vi "WPI_SPIBusCache.vi"(7 "Operation":T2, 8 "error in (no error)":errorcluster, 11 "SPI Bus":T1) -> (0 "error out":errorcluster, 2 "Allocated?":bool, 3 "SPI Bus Allocated":T1)   [LabVIEW 2017]
doc: "This software is licensed. Open the labview\\readme\\WPI Robotics Library Open Source License.txt file for more information."
uses:
  <vilib>/Rock Robotics/WPI/SPI/WPI_SPIBusCacheOp.ctl
  <vilib>/Rock Robotics/SystemInterfaces/spilib/spi_bus.ctl
  <vilib>/Rock Robotics/WPI/PWM/WPI_PWMChannelCacheOp.ctl
  <vilib>/Rock Robotics/WPI/MXP/WPI_MXP SPI Bus to first MXP Pin.vi
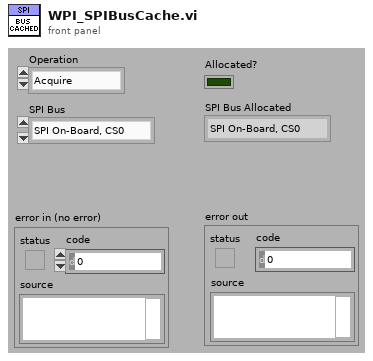
[diagram p1: front panel]
types:
  T1 = typedef "spi_bus.ctl" = enum16{"SPI On-Board, CS0", "SPI On-Board, CS1", "SPI On-Board, CS2", "SPI On-Board, CS3", "SPI MXP", "Invalid"}
  T2 = typedef "WPI_SPIBusCacheOp.ctl" = enum16{"Acquire", "Release", "Status"}
  T3 = typedef "WPI_PWMChannelCacheOp.ctl" = enum16{"Acquire", "Release", "Status"}
  T4 = typedef "WPI_MXP Shared MXP Pin.ctl" = enum16{"11", "13", "15", "17", "19", "21", "23", "25", "27", "29", "31", "18", "22", "26", "32", "34", "Invalid"}
  T5 = typedef "Semaphore RefNum" = refnum<k1>
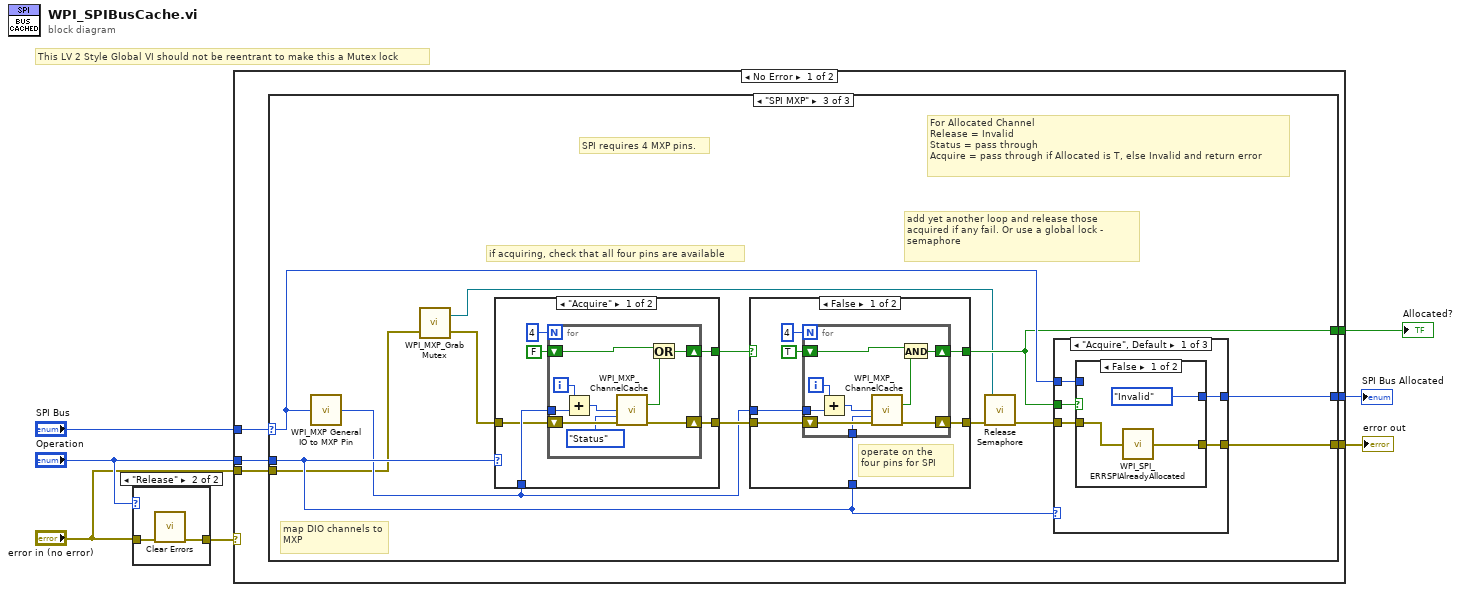
[diagram p0: block diagram]
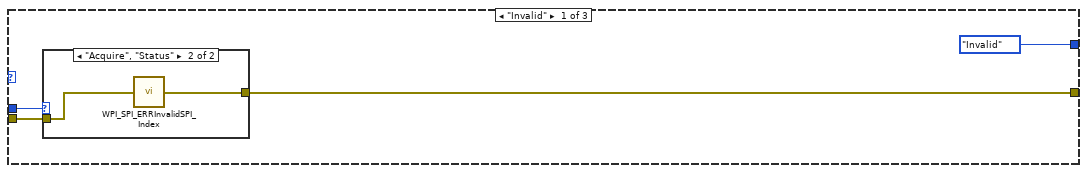
[diagram p3: hidden frame]
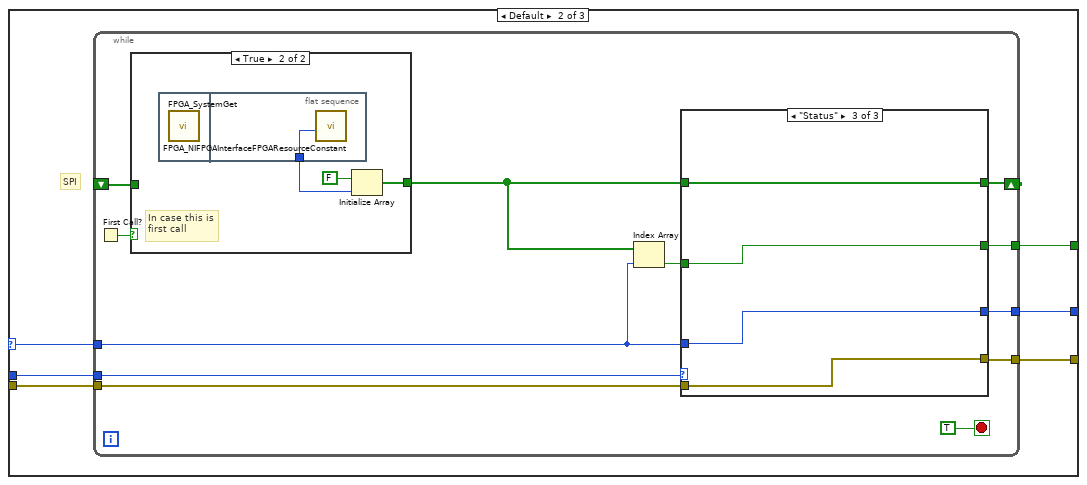
[diagram p5: hidden frame]
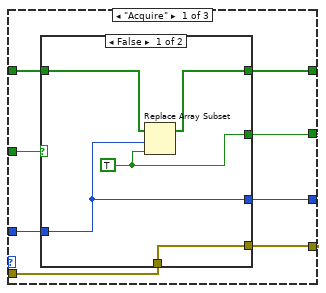
[diagram p6: hidden frame]
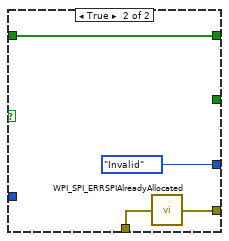
[diagram p7: hidden frame]
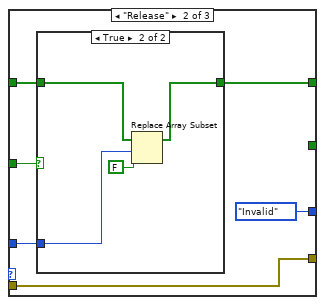
[diagram p8: hidden frame]
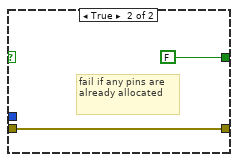
[diagram p11: hidden frame]
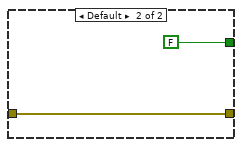
[diagram p12: hidden frame]
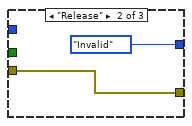
[diagram p14: hidden frame]
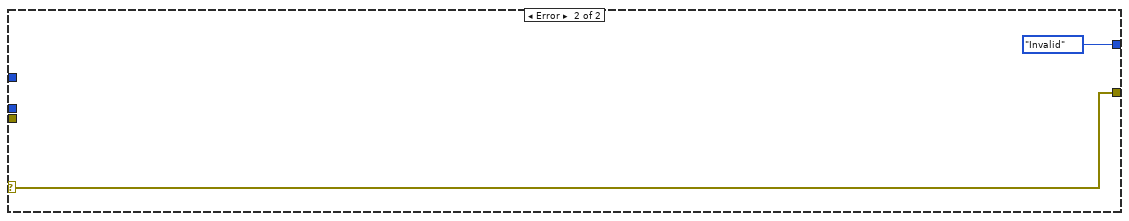
[diagram p16: hidden frame]
diagram:
  # "This LV 2 Style Global VI should not be reentrant to make this a Mutex lock"
  n1 = case shown="\"Release\"" "Operation" {
    tunnel: "error in (no error)" -> [w8 w10]
    tunnel: [w8 w9] -> w4
    frame "Acquire", Default {
    }
    frame "Release" {
      n2 = call <vilib>:"Clear Errors.vi"("error in (no error)"=w10) -> ("error out"=w9:errorcluster)  [unwired: 1 in, 5 out]
    }
  }
  n3 = case shown="No Error" w4 {
    selector: w4 -> [_ w142]
    tunnel: "Operation" -> [w16 _]
    tunnel: "SPI Bus" -> [w15 _]
    tunnel: [w14 w142] -> w1
    tunnel: [w13 _] -> w6
    tunnel: [w12 spi_bus."Invalid" ("SPI Bus")] -> w3
    tunnel: "error in (no error)" -> [w11 _]
    frame No Error {
      n4 = case shown="\"SPI MXP\"" w15 {
        selector: w15 -> [_ w25 w89]
        tunnel: w16 -> [w20 w29 w86]
        tunnel: [w19 w28 w91] -> w14
        tunnel: [_ w27 w85] -> w13
        tunnel: [spi_bus."Invalid" ("SPI Bus") w26 w90] -> w12
        tunnel: w11 -> [w18 w24 w79]
        frame "Invalid" {
          n5 = case shown="\"Acquire\", \"Status\"" w20 {
            tunnel: [w21 w23] -> w19
            tunnel: w18 -> [w21 w22]
            frame "Release" {
            }
            frame "Acquire", "Status" {
              n6 = call <vilib>:"WPI_SPI_ERRInvalidSPI_Index.vi"("error in (no error)"=w22) -> ("error out"=w23:errorcluster)
            }
          }
        }
        frame Default {
          # "SPI"
          n7 = while {
            shift-right: [w38] -> _
            shift-left: _ -> [w40]
            tunnel: w29 -> [w39]
            tunnel: w25 -> [w34]
            tunnel: [w37] -> w28
            tunnel: [w36] -> w27
            tunnel: [w33] -> w26
            tunnel: w24 -> [w31]
            stop <- TRUE stop-if-true
            n8 = First Call?() -> (First Call?: T/F=w41:bool)
            n9 = case shown="True" w41 {
              tunnel: w40 -> [w74 _]
              tunnel: [w74 w77] -> w35
              frame False {
              }
              frame True {
                # "In case this is\nfirst call"
                n10 = flat-sequence {
                  tunnel: [w78] -> w75
                  frame #0 {
                    n11 = call <vilib>:"FPGA_SystemGet.vi"() -> ()  [unwired: 11 in, 1 out]
                  }
                  frame #1 {
                    n12 = call <vilib>:"FPGA_NIFPGAInterfaceFPGAResourceConstant.vi"() -> ("NumberOfSPI"=w78:i32)  [unwired: 11 out]
                  }
                }
                n13 = Initialize Array(FALSE, w75) -> (w77:bool[])
              }
            }
            n14 = Index Array(array=w35, index=w34) -> (element=w30:bool)
            n15 = case shown="\"Status\"" w39 {
              tunnel: w35 -> [w45 w64 w73]
              tunnel: [w49 w62 w73] -> w38
              tunnel: w34 -> [w48 w63 w71]
              tunnel: [w47 w60 w70] -> w37
              tunnel: [w46 _ w72] -> w36
              tunnel: w30 -> [w44 w61 w72]
              tunnel: [w43 spi_bus."Invalid" ("SPI Bus") w71] -> w33
              tunnel: w31 -> [w42 w60 w70]
              frame "Acquire" {
                n16 = case shown="False" w44 {
                  tunnel: w45 -> [w53 w58]
                  tunnel: [w52 w58] -> w49
                  tunnel: w48 -> [w51 _]
                  tunnel: [w50 w57] -> w47
                  tunnel: [w54 _] -> w46
                  tunnel: [w51 spi_bus."Invalid" ("SPI Bus")] -> w43
                  tunnel: w42 -> [w50 w56]
                  frame False {
                    w54 = TRUE ("new element/subarray")
                    n17 = Replace Array Subset(array=w53, new element=w54, index=w51) -> (w52:bool[])
                  }
                  frame True {
                    n18 = call <vilib>:"WPI_SPI_ERRSPIAlreadyAllocated.vi"("error in (no error)"=w56) -> ("error out"=w57:errorcluster)
                  }
                }
              }
              frame "Release" {
                n19 = case shown="True" w61 {
                  tunnel: w64 -> [w65 w69]
                  tunnel: w63 -> [_ w68]
                  tunnel: [w65 w67] -> w62
                  frame False {
                  }
                  frame True {
                    n20 = Replace Array Subset(array=w69, new element=FALSE ("new element/subarray"), index=w68) -> (w67:bool[])
                  }
                }
              }
              frame "Status" {
              }
            }
          }
        }
        frame "SPI MXP" {
          # "add yet another loop and release those acquired if any fail. Or use a global lock - semaphore"
          # "SPI requires 4 MXP pins."
          # "if acquiring, check that all four pins are available"
          # "map DIO channels to MXP"
          # "For Allocated Channel\nRelease = Invalid\nStatus = pass through\nAcquire = pass through if Allocated is T, else Invalid and return error"
          n21 = call-poly <vilib>:"WPI_MXP General IO to MXP Pin.vi"("SPI Bus"=w89) -> ("Shared MXP Pin"=w82:T4)  [unwired: 14 in]
          n22 = call <vilib>:"WPI_MXP_Grab Mutex.vi"("error in"=w79) -> ("error out"=w80:errorcluster, "semaphore out"=w81:T5)  [unwired: 1 in]
          n23 = case shown="\"Acquire\"" w86 {
            tunnel: [w115 w126] -> w88
            tunnel: w82 -> [w114 _]
            tunnel: w80 -> [w113 w126]
            tunnel: [w110 FALSE] -> w87
            frame "Acquire" {
              n24 = for {
                N: 4 -> [_]
                tunnel: w114 -> [w123]
                shift-right: [w124] -> w115
                shift-left: w113 -> [w122]
                shift-right: [w119] -> w110
                shift-left: FALSE -> [w118]
                i -> [w120]
                n25 = Add(x=w120, y=w123) -> (x+y=w121:i32)
                n26 = call <vilib>:"WPI_MXP_ChannelCache.vi"("Shared MXP Pin"=w121, "Operation"=WPI_PWMChannelCacheOp."Status", "error in (no error)"=w122) -> ("Allocated?"=w117:bool, "error out"=w124:errorcluster)  [unwired: 11 in]
                n27 = Or(x=w118, y=w117) -> (x .or. y?=w119:bool)
              }
            }
            frame Default {
            }
          }
          n28 = case shown="False" w87 {
            tunnel: [w98 w109] -> w84
            tunnel: w82 -> [w97 _]
            tunnel: w88 -> [w96 w109]
            tunnel: [w93 FALSE] -> w85
            tunnel: w86 -> [w92 _]
            frame False {
              # "operate on the four pins for SPI"
              n29 = for {
                N: 4 -> [_]
                tunnel: w97 -> [w106]
                shift-right: [w107] -> w98
                shift-left: w96 -> [w105]
                shift-right: [w102] -> w93
                shift-left: TRUE -> [w101]
                tunnel: w92 -> [w99]
                i -> [w103]
                n30 = Add(x=w103, y=w106) -> (x+y=w104:i32)
                n31 = call <vilib>:"WPI_MXP_ChannelCache.vi"("Shared MXP Pin"=w104, "Operation"=w99, "error in (no error)"=w105) -> ("Allocated?"=w100:bool, "error out"=w107:errorcluster)  [unwired: 11 in]
                n32 = And(x=w101, y=w100) -> (x .and. y?=w102:bool)
              }
            }
            frame True {
              # "fail if any pins are already allocated"
            }
          }
          n33 = call <vilib>:"Release Semaphore.vi"("error in (no error)"=w84, "semaphore"=w81) -> ("error out"=w83:errorcluster)  [unwired: 4 in, 1 out]
          n34 = case shown="\"Acquire\", Default" w86 {
            tunnel: [w130 spi_bus."Invalid" ("SPI Bus") w140] -> w90
            tunnel: w89 -> [w129 _ w140]
            tunnel: w83 -> [w128 w138 w139]
            tunnel: w85 -> [w131 _ _]
            tunnel: [w127 w138 w139] -> w91
            frame "Acquire", Default {
              n35 = case shown="False" w131 {
                tunnel: [spi_bus."Invalid" ("SPI Bus") w136] -> w130
                tunnel: w129 -> [_ w136]
                tunnel: w128 -> [w132 w135]
                tunnel: [w134 w135] -> w127
                frame False {
                  n36 = call <vilib>:"WPI_SPI_ERRSPIAlreadyAllocated.vi"("error in (no error)"=w132) -> ("error out"=w134:errorcluster)
                }
                frame True {
                }
              }
            }
            frame "Release" {
            }
            frame "Status" {
            }
          }
        }
      }
    }
    frame Error {
    }
  }
  "Allocated?" <- w6
  "error out" <- w1
  "SPI Bus Allocated" <- w3
